vi "templates create js data.vi"(5 "Changes?":bool, 6 "sxUsername":string, 7 "POST Parameters":T1, 8 "error in (no error)":errorcluster, 9 "template Parameters":T1, 10 "Template Record":T3, 11 "Connection Refnum":T2) -> (0 "error out":errorcluster, 2 "HTM Keys":T1, 3 "Connection Refnum":T2)   [LabVIEW 2011]
uses:
  Addons/internet/utils/keyedarr.llb/Keyed Array.ctl
  server/database/Templates/Template Record.ctl
  SI.LIB/ODBC/SQL Controls/Connection Refnum.ctl
  Addons/internet/utils/strutil.llb/Case Matching.ctl
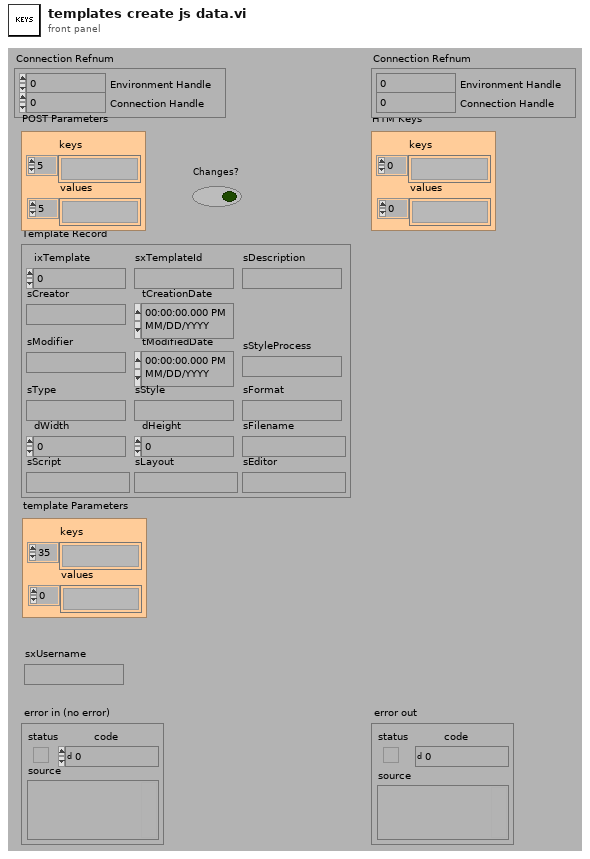
[diagram p1: front panel]
types:
  T1 = typedef "Keyed Array.ctl" = cluster{"keys":string[], "values":string[]}
  T2 = typedef "Connection Refnum.ctl" = cluster{"Environment Handle":i32, "Connection Handle":i32}
  T3 = typedef "Template Record.ctl" = cluster{"ixTemplate":i32, "sxTemplateId":string, "sDescription":string, "sCreator":string, "tCreationDate":timestamp, "sModifier":string, "tModifiedDate":timestamp, "sType":string, "sStyle":string, "sFormat":string, "dWidth":dbl, "dHeight":dbl, "sFilename":string, "sScript":string, "sLayout":string, "sEditor":string, "sStyleProcess":string}
  T4 = typedef "Case Matching.ctl" = enum16{"a != A", "a == A", "system"}
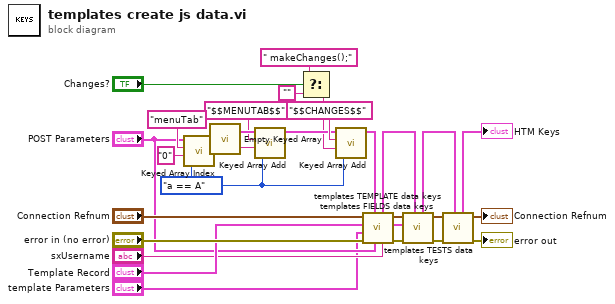
[diagram p0: block diagram]
diagram:
  w1 = Case_Matching."a == A" ("case matching (sensitive)")
  n1 = call "Keyed Array Index.vi"("case matching (sensitive)"=w1, "default value"="0", "key"="menuTab", "array in"="POST Parameters") -> ("value"=w13:string)  [unwired: 3 out]
  n2 = call "Empty Keyed Array.vi"() -> ("empty keyed array"=w14:T1)  [unwired: 3 out]
  n3 = call "Keyed Array Add.vi"("case matching (sensitive)"=w1, "value"=w13, "key"="$$MENUTAB$$", "array in"=w14) -> ("array out"=w7:T1)  [unwired: 3 out]
  n4 = Select(t=" makeChanges();" ("key"), s="Changes?", f="") -> (s? t:f=w2:string)
  n5 = call "Keyed Array Add.vi"("case matching (sensitive)"=w1, "value"=w2, "key"="$$CHANGES$$", "array in"=w7) -> ("array out"=w6:T1)  [unwired: 3 out]
  n6 = call "templates TEMPLATE data keys.vi"("sxUsername"="sxUsername", "POST Parameters"="POST Parameters", "HTM Keys"=w6, "error in (no error)"="error in (no error)", "Template Parameters"="template Parameters", "Template Record"="Template Record", "Connection Refnum"="Connection Refnum") -> ("error out"=w26:errorcluster, "Template Keys"=w17:T1, "Connection Refnum"=w25:T2, "HTM Keys"=w24:T1)  [unwired: 1 out]
  n7 = call "templates FIELDS data keys.vi"("HTM Keys"=w24, "error in (no error)"=w26, "Template Keys"=w17, "Connection Refnum"=w25) -> ("error out"=w23:errorcluster, "Connection Refnum"=w20:T2, "HTM Keys"=w18:T1)  [unwired: 5 out]
  n8 = call "templates TESTS data keys.vi"("HTM Keys"=w18, "error in (no error)"=w23, "Connection Refnum"=w20) -> ("error out"=→"error out":errorcluster, "Connection Refnum"=→"Connection Refnum":T2, "HTM Keys"=→"HTM Keys":T1)  [unwired: 6 out]
